vi "Analog Output DAQ.vi"() -> ()   [LabVIEW 2020]
panel:
  out "Waveform Graph":dynamicdata(graph)
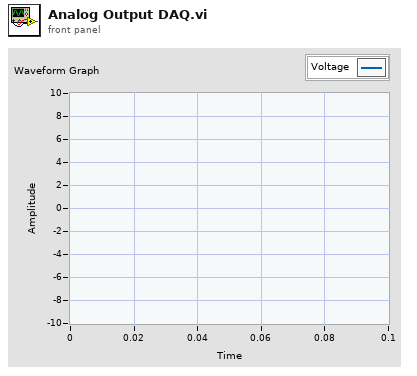
[diagram p1: front panel]
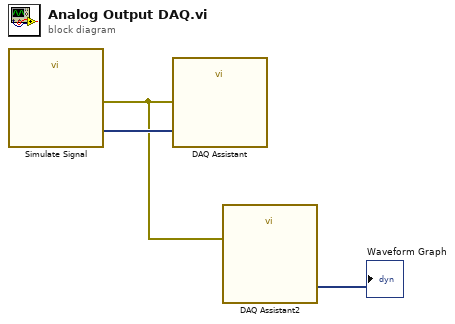
[diagram p0: block diagram]
diagram:
  n1 = call "Simulate Signal"() -> ("Sine"=w3:dynamicdata, "error out"=w1:errorcluster)  [unwired: 14 in]
  n2 = call "DAQ Assistant"("data"=w3, "error in"=w1) -> ()  [unwired: 16 in, 2 out]
  n3 = call "DAQ Assistant2"("error in"=w1) -> ("data"=→"Waveform Graph":dynamicdata)  [unwired: 16 in, 2 out]
